vi "Write History Length.vi"(8 "Error In":errorcluster, 10 "History Length":u32, 11 "History Length Msg":refnum<class "History Length Msg.lvclass">) -> (0 "Error Out":errorcluster, 3 "History Length Msg":refnum<class "History Length Msg.lvclass">)   [LabVIEW 2019, in "BNT_XtGraph.lvlib" / "History Length Msg.lvclass"]
uses:
  History Length Msg.lvclass
  History Length Msg.lvclass/History Length Msg.ctl
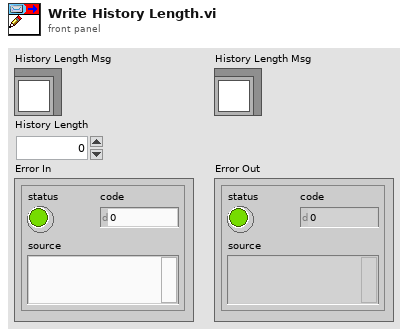
[diagram p1: front panel]
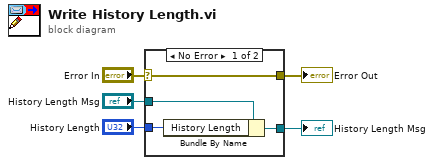
[diagram p0: block diagram]
diagram:
  n1 = case shown="No Error" "Error In" {
    selector: "Error In" -> [w9 w10]
    tunnel: [w9 w10] -> w5
    tunnel: [w7 w11] -> w3
    tunnel: "History Length Msg" -> [w8 w11]
    tunnel: "History Length" -> [w6 _]
    frame No Error {
      n2 = Bundle By Name(cluster=w8, "History Length"=w6) -> (w7:refnum<class "History Length Msg.lvclass">)
    }
    frame Error {
    }
  }
  "History Length Msg" <- w3
  "Error Out" <- w5
